vi "Height Suggestion.vi"(7 "array":dbl[](array[numeric]), 8 "Droplet Size":dbl, 9 "Input Voltage":dbl, 10 "Initial Charge":dbl, 11 "Evaporation Time":dbl) -> (3 "Suggested Height":dbl)   [LabVIEW 2020]
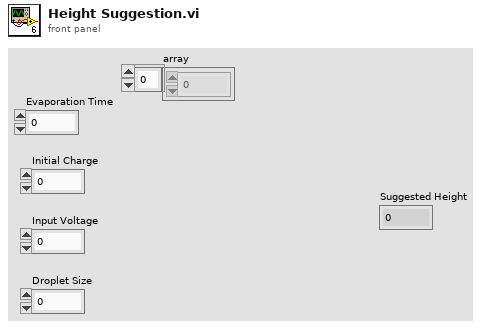
[diagram p1: front panel]
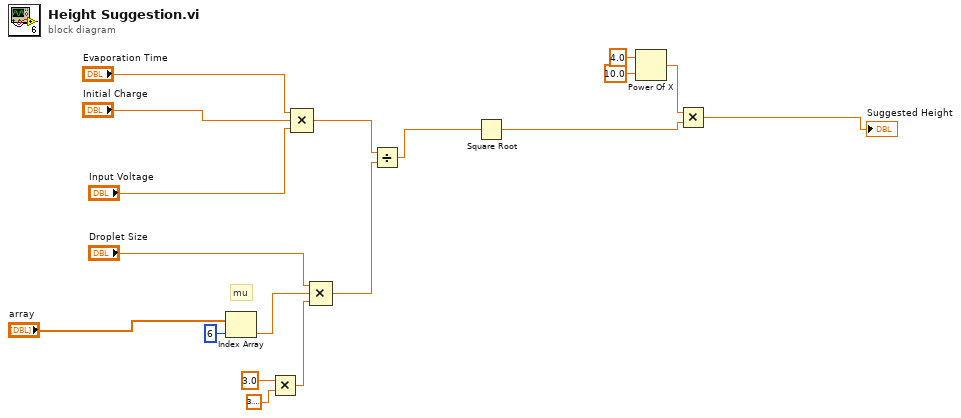
[diagram p0: block diagram]
diagram:
  # "mu"
  n1 = Index Array(array="array", index=6) -> (element=w13:dbl)
  n2 = Multiply(x=3.0, y=3.141592653589793) -> (x*y=w12:dbl)
  n3 = Compound Arithmetic op=MULTIPLY("Evaporation Time", "Initial Charge", "Input Voltage") -> (w9:dbl)
  n4 = Compound Arithmetic op=MULTIPLY("Droplet Size", w13, w12) -> (w8:dbl)
  n5 = Divide(x=w9, y=w8) -> (x/y=w7:dbl)
  n6 = Square Root(x=w7) -> (sqrt(x)=w5:dbl)
  n7 = Power Of X(1:10.0 ("x"), 2:4.0 ("y")) -> (0:w2:dbl)
  n8 = Multiply(x=w2, y=w5) -> (x*y=→"Suggested Height":dbl)
